vi "availableDAQ.vi"(8 "error in (no error)":errorcluster) -> (0 "error out":errorcluster, 3 "DAQmx Device Name":tag)   [LabVIEW 2013, in "main.lvlib"]
uses:
  main.lvlib
  <resource>/objmgr/daqmx.rc
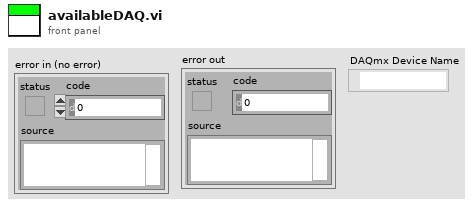
[diagram p1: front panel]
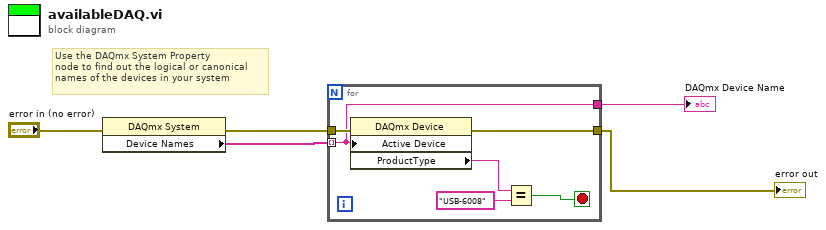
[diagram p0: block diagram]
diagram:
  # "Use the DAQmx System Property\nnode to find out the logical or canonical\nnames of the devices in your system"
  n1 = property class="DAQmx System"(error in="error in (no error)") -> (error out=w3:errorcluster, "Device Names"=w2:tag[])  [unwired: 1 in, 1 out]
  n2 = for {
    tunnel: w2 -> [w6] mode=indexing
    tunnel: w3 -> [w11]
    tunnel: [w10] -> w4
    tunnel: [w6] -> w5
    stop <- w7 stop-if-true
    n3 = property class="DAQmx Device"(error in=w11, "Active Device"=w6) -> (error out=w10:errorcluster, "ProductType"=w9:string)  [unwired: 1 in, 1 out]
    n4 = Equal?(x=w9, y="USB-6008") -> (x = y?=w7:bool)
  }
  "error out" <- w4
  "DAQmx Device Name" <- w5
